vi "SRX_Fill Motion Buffer.vi"(7 "Profile Array":T7[](array[typedef]), 8 "Error":errorcluster, 10 "Motion Buffer Status":T1, 11 "SingleMotorRef":T2={"DeviceStatus"={"status"=FALSE, "code"=0, "source"=""}, "Type"=enum."PWM", "PWM"={"PWM Channel"=enum."PWM 0", "DeadBand"={"Name"="", "maxPositivePwm"=0, "minPositivePwm"=0, "centerPwm"=0, "maxNegativePwm"=0, "minNegativePwm"=0, "angularRange"=0}}, "CAN"={"Device Number"=0, "SetOutput VI Ref"=variant, "GetOutput VI Ref"=variant, "Enable VI Ref"=variant, "Disable VI Ref"=variant, "Data"=variant}, "Invert"=FALSE, "DIO PWM"={"PWM \"Enable\" Channel"=enum."Invalid", "DIOChannel"=enum."Invalid", "PWM Rate"=0.0}}) -> (0 "Error Out":errorcluster, 2 "Motion Buffer Status Out":T1, 3 "SingleMotorRef Out":T2={"DeviceStatus"={"status"=FALSE, "code"=0, "source"=""}, "Type"=enum."PWM", "PWM"={"PWM Channel"=enum."PWM 0", "DeadBand"={"Name"="", "maxPositivePwm"=0, "minPositivePwm"=0, "centerPwm"=0, "maxNegativePwm"=0, "minNegativePwm"=0, "angularRange"=0}}, "CAN"={"Device Number"=0, "SetOutput VI Ref"=variant, "GetOutput VI Ref"=variant, "Enable VI Ref"=variant, "Disable VI Ref"=variant, "Data"=variant}, "Invert"=FALSE, "DIO PWM"={"PWM \"Enable\" Channel"=enum."Invalid", "DIOChannel"=enum."Invalid", "PWM Rate"=0.0}}, 5 "Buffer Full Out":bool)   [LabVIEW 2017]
uses:
  <vilib>/Rock Robotics/WPI/MotorControl/WPI_MotorControlDeviceRef.ctl
  <vilib>/Rock Robotics/WPI/MotorControl/WPI_MotorControlType.ctl
  <vilib>/Rock Robotics/SystemInterfaces/DIO/FPGA_DIOPWMChannel.ctl
  <vilib>/Rock Robotics/WPI/PWM/WPI_PWMDeadband.ctl
  <vilib>/Rock Robotics/SystemInterfaces/DIO/FPGA_DIOChannel.ctl
  TypeDef/CLUSTER_Drive_Point Specification.ctl
  TypeDef/ENUM_Drive_SRX Motion Buffer Status.ctl
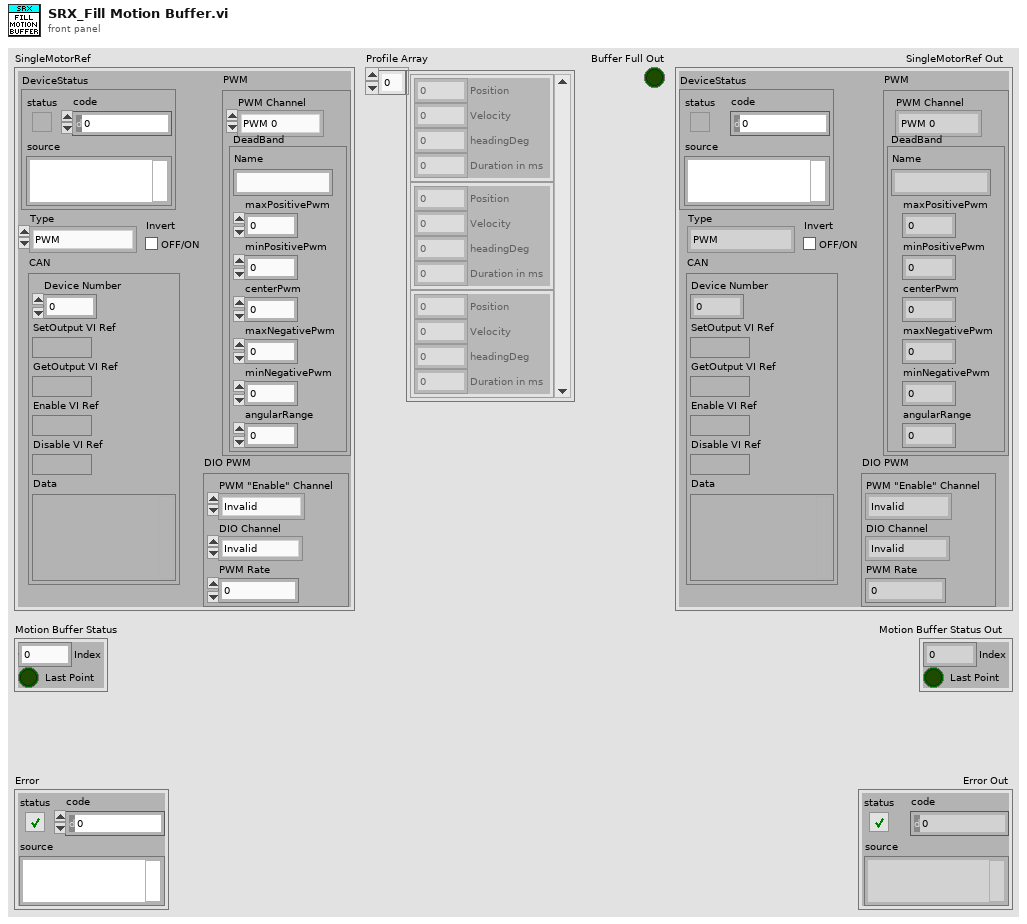
[diagram p1: front panel]
types:
  T1 = typedef "ENUM_Drive_SRX Motion Buffer Status.ctl" = cluster{"Index":i32, "Last Point":bool}
  T2 = typedef "WPI_MotorControlDeviceRef.ctl" = cluster{"DeviceStatus":errorcluster, "Type":T3, "PWM":cluster{"PWM Channel":T4, "DeadBand":T5}, "CAN":cluster{"Device Number":u8, "SetOutput VI Ref":variant, "GetOutput VI Ref":variant, "Enable VI Ref":variant, "Disable VI Ref":variant, "Data":variant}, "Invert":bool, "DIO PWM":cluster{"PWM \"Enable\" Channel":T4, "DIOChannel":T6, "PWM Rate":dbl}}
  T3 = typedef "WPI_MotorControlType.ctl" = enum16{"PWM", "CAN", "DIO PWM"}
  T4 = typedef "FPGA_DIOPWMChannel.ctl" = enum8{"PWM 0", "PWM 1", "PWM 2", "PWM 3", "PWM 4", "PWM 5", "PWM 6", "PWM 7", "PWM 8", "PWM 9", "PWM MXP 0", "PWM MXP 1", "PWM MXP 2", "PWM MXP 3", "PWM MXP 4", "PWM MXP 5", "PWM MXP 6", "PWM MXP 7", "PWM MXP 8", "PWM MXP 9", "Invalid"}
  T5 = typedef "WPI_PWMDeadband.ctl" = cluster{"Name":string, "maxPositivePwm":i32, "minPositivePwm":i32, "centerPwm":i32, "maxNegativePwm":i32, "minNegativePwm":i32, "angularRange":u16}
  T6 = typedef "FPGA_DIOChannel.ctl" = enum8{"DIO 0", "DIO 1", "DIO 2", "DIO 3", "DIO 4", "DIO 5", "DIO 6", "DIO 7", "DIO 8", "DIO 9", "DIO MXP 0", "DIO MXP 1", "DIO MXP 2", "DIO MXP 3", "DIO MXP 4", "DIO MXP 5", "DIO MXP 6", "DIO MXP 7", "DIO MXP 8", "DIO MXP 9", "DIO MXP 10", "DIO MXP 11", "DIO MXP 12", "DIO MXP 13", "DIO MXP 14", "DIO MXP 15", "SPI Port CS1", "SPI Port CS2", "SPI Port CS3", "SPI Port MISO", "SPI Port MOSI", "Invalid"}
  T7 = typedef "CLUSTER_Drive_Point Specification.ctl" = cluster{"Position":dbl, "Velocity":dbl, "headingDeg":dbl, "Duration in ms":i32}
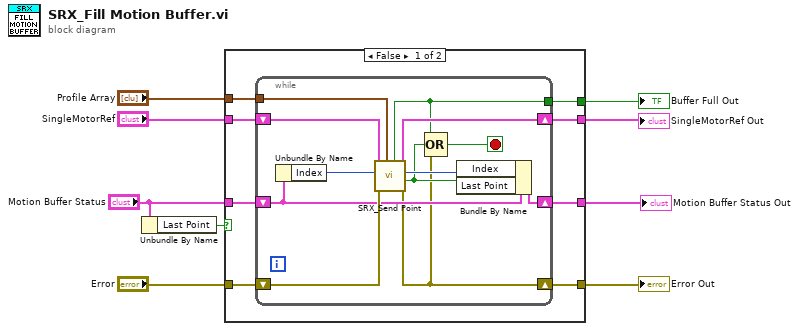
[diagram p0: block diagram]
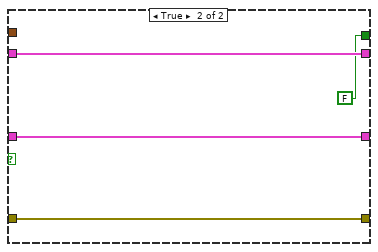
[diagram p2: hidden frame]
diagram:
  n1 = Unbundle By Name("Motion Buffer Status") -> ("Last Point"=w1:bool)
  n2 = case shown="False" w1 {
    tunnel: "SingleMotorRef" -> [w17 w33]
    tunnel: "Profile Array" -> [w16 _]
    tunnel: [w15 w33] -> w7
    tunnel: "Error" -> [w14 w30]
    tunnel: [w13 w30] -> w5
    tunnel: [w12 FALSE ("Buffer Full Out")] -> w4
    tunnel: [w11 w31] -> w3
    tunnel: "Motion Buffer Status" -> [w10 w31]
    frame False {
      n3 = while {
        tunnel: w16 -> [w28]
        tunnel: [w24] -> w12
        shift-right: [w21] -> w11
        shift-left: w10 -> [w22]
        shift-right: [w27] -> w15
        shift-left: w17 -> [w29]
        shift-right: [w18] -> w13
        shift-left: w14 -> [w26]
        stop <- w25 stop-if-true
        n4 = Unbundle By Name(w22) -> ("Index"=w23:i32)
        n5 = call "SRX_Send Point.vi"("Point Array"=w28, "Error"=w26, "Index"=w23, "CAN Talon SRX Ref"=w29) -> ("Error Out"=w18:errorcluster, "Last Point Out"=w19:bool, "Next Index Out"=w20:i32, "CAN Talon SRX Ref Out"=w27:T2, "Buffer Full Out"=w24:bool)  [unwired: 3 in]
        n6 = Compound Arithmetic op=OR(w24, w19, w18) -> (w25:bool)
        n7 = Bundle By Name(cluster=w22, "Index"=w20, "Last Point"=w19) -> (w21:T1)
      }
    }
    frame True {
    }
  }
  "SingleMotorRef Out" <- w7
  "Error Out" <- w5
  "Buffer Full Out" <- w4
  "Motion Buffer Status Out" <- w3
